vi "create.vi"(8 "error in":errorcluster, 10 "size (1,10000)":i32=1000) -> (0 "error out":errorcluster, 3 "message connection out":refnum<class "identifying queue.lvclass">)   [LabVIEW 2015, in "identifying queue.lvclass"]
uses:
  identifying queue.lvclass
  message/communicator message.lvclass
  identifying queue.lvclass/identifying queue.ctl
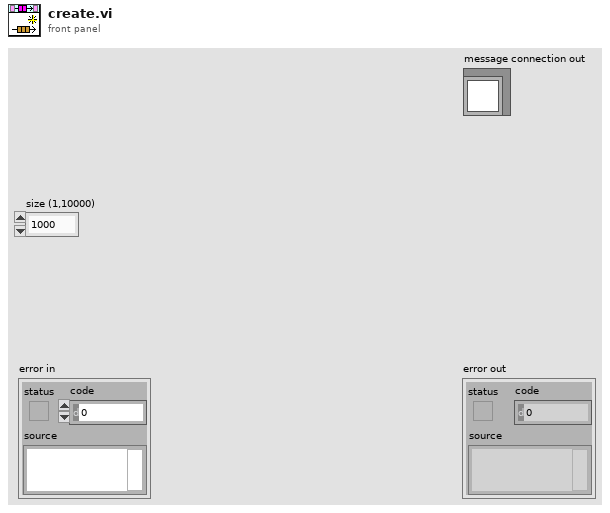
[diagram p1: front panel]
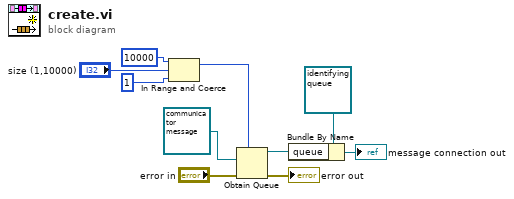
[diagram p0: block diagram]
diagram:
  n1 = In Range and Coerce(upper limit=10000, x="size (1,10000)", lower limit=1) -> (coerced(x)=w4:i32)  [unwired: 1 out]
  n2 = Obtain Queue(max queue size (-1, unlimited)=w4, element data type=refnum<class "communicator message.lvclass"> refnum ("communicator message.lvclass"), error in (no error)="error in") -> (queue out=w1:refnum<queue>, error out=→"error out":errorcluster)  [unwired: 2 in, 1 out]
  n3 = Bundle By Name(cluster=refnum<class "identifying queue.lvclass"> refnum ("message connection out"), "queue"=w1) -> (→"message connection out":refnum<class "identifying queue.lvclass">)
